vi "Parse-Sort-Split.vi"(5 "AE Groups":T1(array[ring])=[enum."AE-Germany", enum."AE-Poland", enum."AE-Switzerland", enum."AE-Czech Republic", enum."AE-Hungary", enum."AE-Romania", enum."AE-Slovakia", enum."AE-Slovenia"], 7 "Include High Priority?":bool, 8 "Error In":errorcluster, 11 "SR List In":T2(array[cluster])) -> (0 "Error Out":errorcluster, 2 "Unassigned SR List":T2(array[cluster]), 3 "Assigned SR List":T2(array[cluster]))   [LabVIEW 2017, in "Client.lvlib"]
uses:
  Client.lvlib
  ParserSorter.lvlib
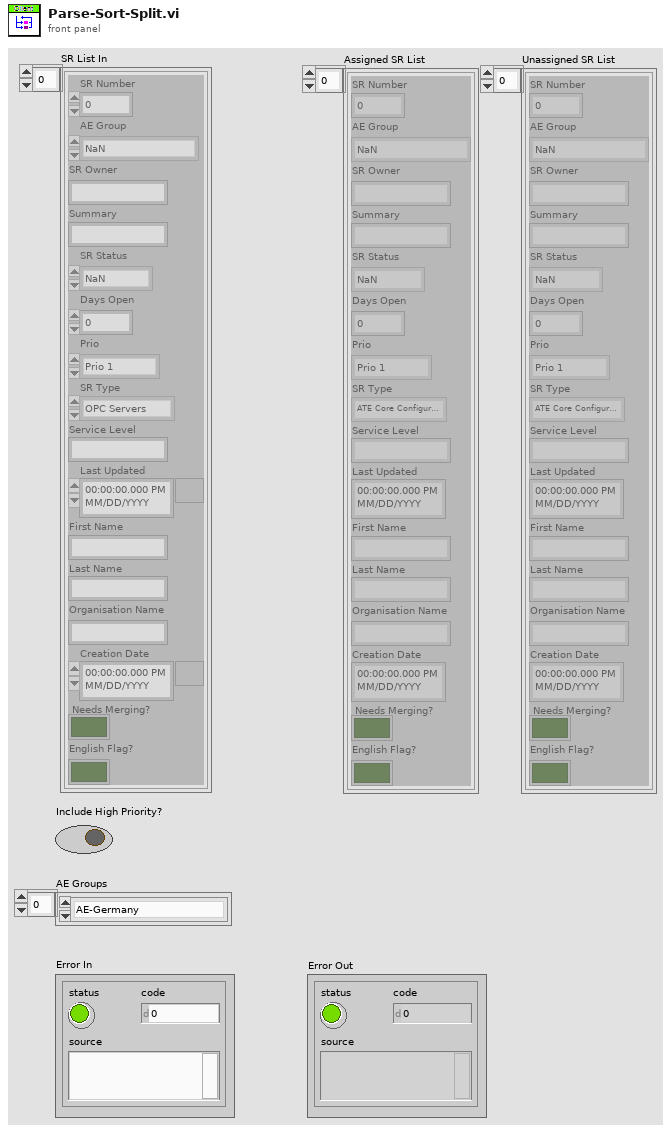
[diagram p1: front panel]
types:
  T1 = enum32{"NaN", "AE-Germany", "AE-Poland", "AE-Switzerland", "AE-Czech Republic", "AE-Hungary", "AE-Romania", "AE-Slovakia", "AE-Slovenia"}[]
  T2 = cluster{"SR Number":i64, "AE Group":enum32{"NaN", "AE-Germany", "AE-Poland", "AE-Switzerland", "AE-Czech Republic", "AE-Hungary", "AE-Romania", "AE-Slovakia", "AE-Slovenia"}, "SR Owner":string, "Summary":string, "SR Status":enum32{"NaN", "Caller Abandoned", "Created in Error", "Declined to Purchase Support", "Expired", "Forum Resolved AE", "Forum Resolved Customer", "IN WORK", "IN WORK Collab with AES", "IN WORK Collab with PSE", "IN WORK Collab with SE", "IN WORK Escalation", "IN WORK Customer Added Note", "Open", "Potentially Resolved", "POC Resolved", "Resolved", "RMA Waiting on Customer", "RMA Open", "RMA In Progress", "RMA Closed - DOA", "RMA Closed", "RMA Approved for Return", "Project Complete", "Presumed Resolved", "IN WORK Wait on Customer"}, "Days Open":dbl, "Prio":enum16{"Prio 1", "Prio 2", "Prio 3", "Prio 4"}, "SR Type":enum32{"NaN", "ATE Core Configurations (BYOATE)", "Activation", "BioBench", "CAN", "CM C Series", "Calibration", "Consulting Services", "CounterTimer", "DAQExpress", "DASYLab", "DIAdem", "DMM", "DSA HW", "Digital_IO", "FIRST (NIC Only)", "FieldBus", "FieldPoint", "Functional Savety", "GATI", "GPIB", "HMI and Industrial PCs", "HiQ", "HighSpeedDigital_IO", "IMAQ", "IOTech Vibration", "Industrial Communications", "InsightCM", "LV", "LV CD&Sim", "LV Comms", "LV Controls Add-Ons", "LV Embedded", "LV MathScript RT", "LV NXG", "LV NXT", "LVDSC", "LVFPGA", "LVPDA and LV Touch Panel", "LVRT", "LabWindows_CVI", "Lookout", "MATRIXx", "MStudioDotNet", "MStudioVisualBasic", "MStudioVisualC", "Measure (Legacy)", "Motion", "MultifunctionDAQ", "Multimedia Test HW/SW", "Multisim (EWB)", "NI Update Service", "OPC Servers", "Optical (OSI)", "PXI Controllers, Chassis, MXI", "PXI Timing and Sync", "Power Supplies and SMUs", "Powertrain Controls", "RAID", "RF", "RF Software", "RIO", "SC Express", "SCC", "SCXI", "SPEEDY-33 (Hyperception)", "STS", "ScopeDigitizers", "Serial", "Signal Sources", "SignalCondOther", "SignalExpress", "Software Defined Intruments", "Sound and Vibration SW", "Switch Executive", "Switches", "TestStand", "USRP", "Ultiboard (EWB)", "VBench", "VI Logger", "VXI_MXI", "VeriStand", "VisionSW", "VolumeLicenseMgr", "WSN", "Web UI Builder", "myRIO"}, "Service Level":string, "Last Updated":timestamp, "First Name":string, "Last Name":string, "Organisation Name":string, "Creation Date":timestamp, "Needs Merging?":bool, "English Flag?":bool}[]
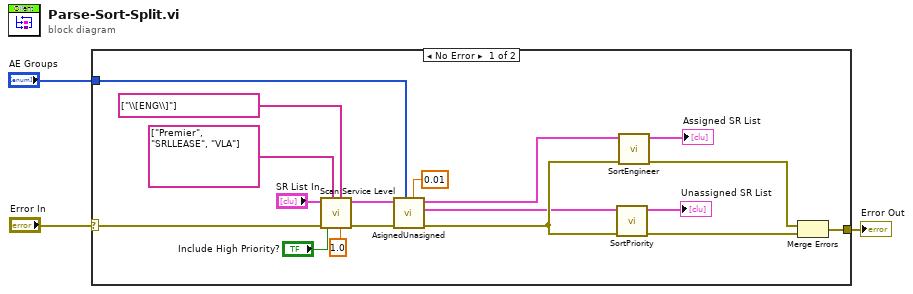
[diagram p0: block diagram]
diagram:
  n1 = case shown="No Error" "Error In" {
    selector: "Error In" -> [w18 w22]
    tunnel: [w10 w22] -> w2
    tunnel: "AE Groups" -> [w4 _]
    frame No Error {
      n2 = call "Scan Service Level.vi"("Days Open Prio Threshold"=1.0, "English Tags"=string[] ["\\[ENG\\]"], "Include High Priority?"="Include High Priority?", "Premier Levels Keywords"=string[] ["Premier", "SRLLEASE", "VLA"], "error in (no error)"=w18, "Array in"="SR List In") -> ("error out"=w17:errorcluster, "Array out"=w16:T2)  [unwired: 4 in]
      n3 = call "AsignedUnasigned.vi"("Days Open Phone Treshhold"=0.01, "AE Groups"=w4, "error in (no error)"=w17, "All SR In"=w16) -> ("error out"=w14:errorcluster, "Unassigned"=w12:T2, "Assigned Out"=w13:T2)  [unwired: 5 in]
      n4 = call "SortPriority.vi"("error in (no error)"=w14, "Array in"=w12) -> ("error out"=w8:errorcluster, "Array out"=→"Unassigned SR List":T2)  [unwired: 8 in]
      n5 = call "SortEngineer.vi"("error in (no error)"=w14, "Array in"=w13) -> ("error out"=w9:errorcluster, "Array out"=→"Assigned SR List":T2)  [unwired: 8 in]
      n6 = Merge Errors(w9, w8) -> (w10:errorcluster)
    }
    frame Error {
    }
  }
  "Error Out" <- w2
